vi "Main.vi"() -> ()   [LabVIEW 2025]
doc: "This template is for the Queued Message Handler design pattern.\n\nThe Event Handling Loop generates messages based on user interface actions.\n\nThe Message Handling Loop processes messages generated by the Event Handling Loop, or by other messages. The messages are string values, so new messages can be added easily to the Message Cases case structure in the Message Handling Loop. Each message cluster can also provide an optional value for Message Data, which is a variant that can be converted to whatever message-specific data is required."
uses:
  controls/UI Data.ctl
  support/Message Queue/Enqueue Message (Single).vi
  <vilib>/Utility/file.llb/Write Delimited Spreadsheet (string).vi
  <vilib>/Utility/error.llb/Error Cluster From Error Code.vi
  <vilib>/ErrorRing/Error Ring.xnode
  support/Message Queue/Message Queue.lvlib
  support/User Event - Stop/User Event - Stop.lvlib
  <instrlib>/BK Precision 9200 Series/BK Precision 9200 Series.lvlib
  <instrlib>/Agilent 34970/Agilent 34970.lvlib
panel:
  out "Table":string[][](table)
  out "Current Cycle":u16
  in  "Total Cycles":u16
  in  "Voltage Channel":string
  out "Connected_RELAY":bool caption="Connected_DAQ"
  in  "RELAY CONTROL":refnum<visa-resource-name>
  out "Connected_DAQ":bool
  in  "DAQ970A":refnum<visa-resource-name>
  out "Connected_ps":bool
  in  "POWER SUPPLY":refnum<visa-resource-name>
  out "DAQ_Amps":dbl format="%#_4fA"
  out "DAQ_Volt":dbl format="%#_4fV"
  out "PS_Amps":dbl format="%#_4fA"
  out "PS_Volt":dbl format="%#_4fV"
  out "Status":string
  in  "Start/Stop":enum32{"Item 0", "Item 1"}(radio)=enum."Item 1"
  in  "Exit":bool
  # "DC-DC Short Circuit Durability"
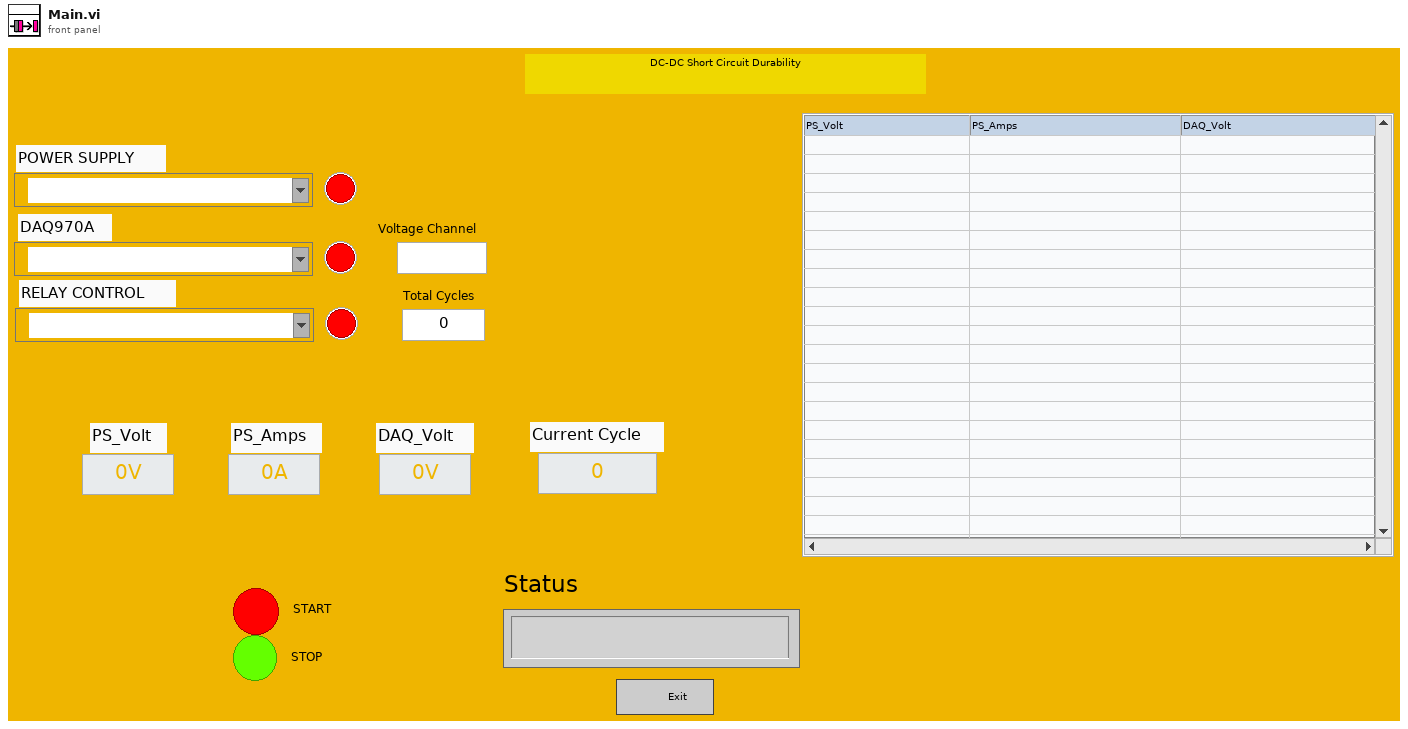
[diagram p1: front panel]
types:
  T1 = typedef "UI Data.ctl" = cluster{"Boolean <Replace Me>":bool, "Status":string, "Cycle Count":u16, "POWER SUPPLY":refnum<visa-resource-name>, "DAQ6510":refnum<visa-resource-name>, "RELAY CONTROL":refnum<visa-resource-name>, "Error Status ":string, "Current Cycle":u16, "Table":string[][], "Data_array":string[], "Started?":bool, "Datapath":path}
  T2 = typedef "Message Queue.lvlib/All Message Queues.ctl" = cluster{"UI":refnum<queue>}
  T3 = enum16{"4 1/2", "5 1/2", "6 1/2", "Least", "Highest", "Default"}
  T4 = cluster{"Timeout Value (10000)":u32, "Baud Rate (57600)":enum16{"1200", "2400", "4800", "9600", "19200", "38400", "57600", "115200"}, "Flow Control (1:XON/XOFF)":enum16{"None", "XON / XOFF", "RTS / CTS", "DTR / DSR"}}
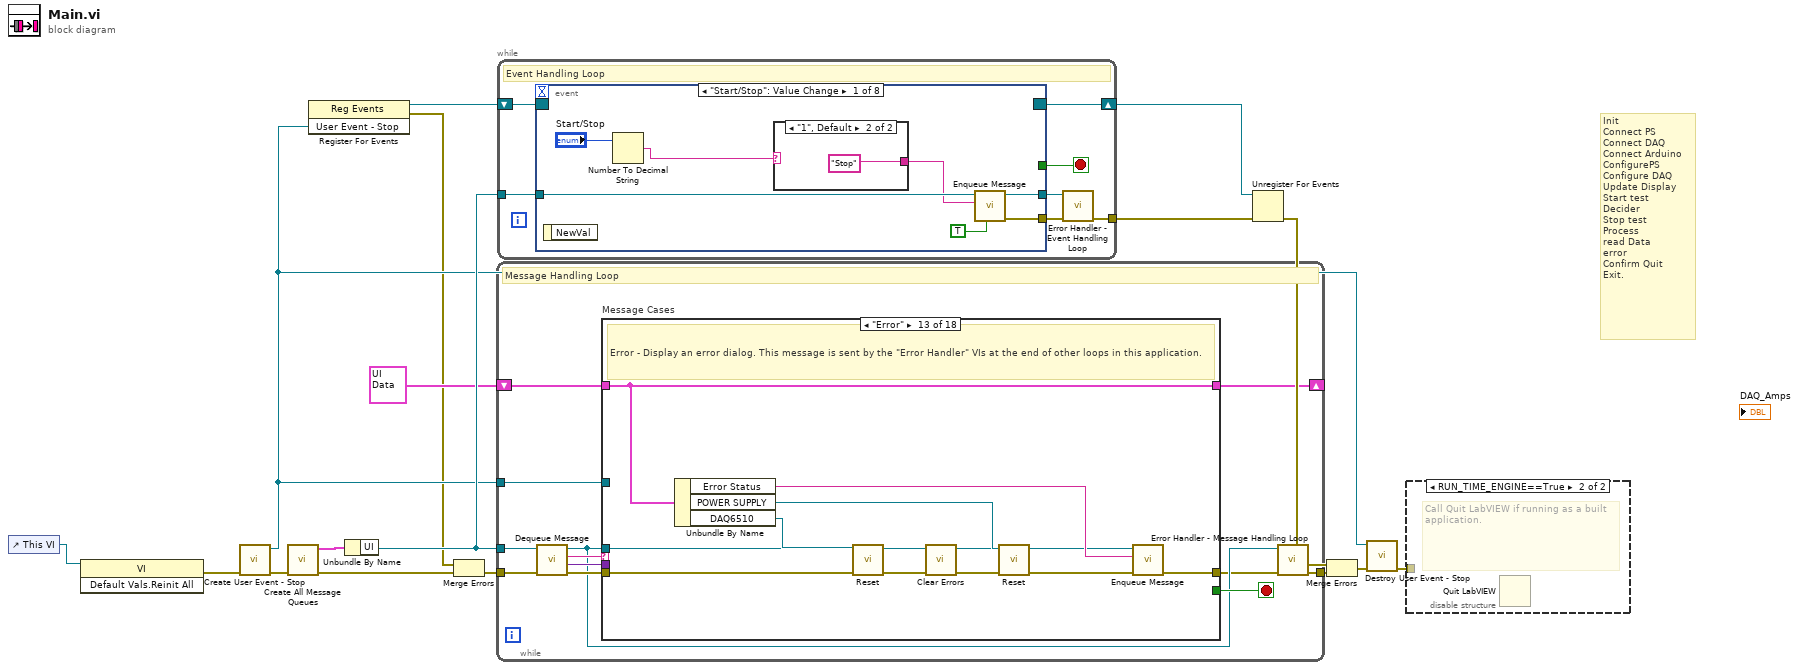
[diagram p0: block diagram]
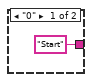
[diagram p3: hidden frame]
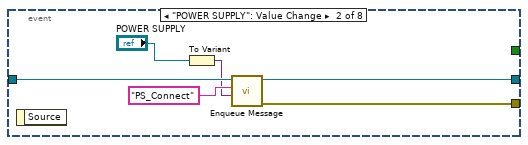
[diagram p4: hidden frame]
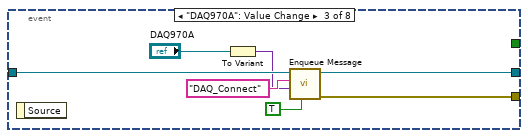
[diagram p5: hidden frame]
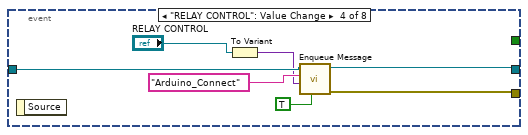
[diagram p6: hidden frame]
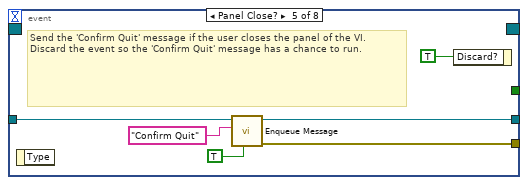
[diagram p7: hidden frame]
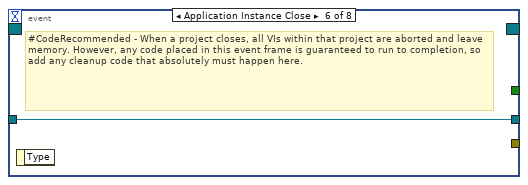
[diagram p8: hidden frame]
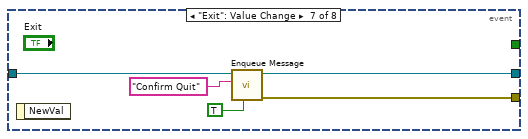
[diagram p9: hidden frame]
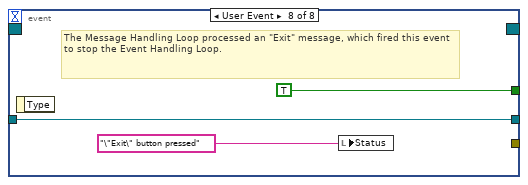
[diagram p10: hidden frame]
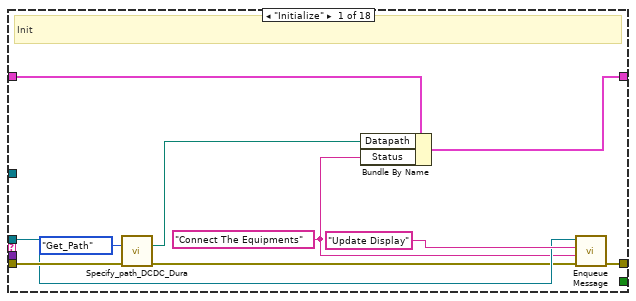
[diagram p11: hidden frame]
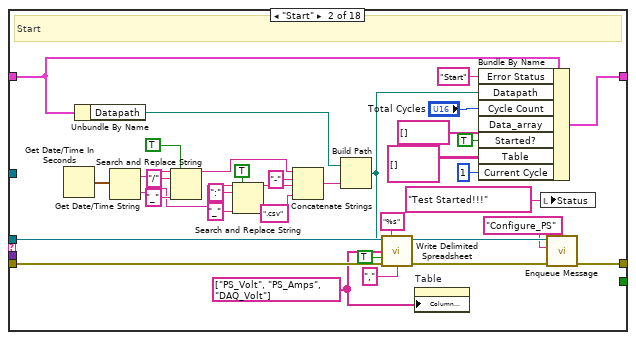
[diagram p12: hidden frame]
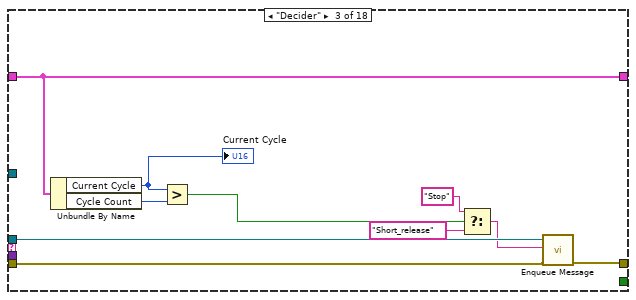
[diagram p13: hidden frame]
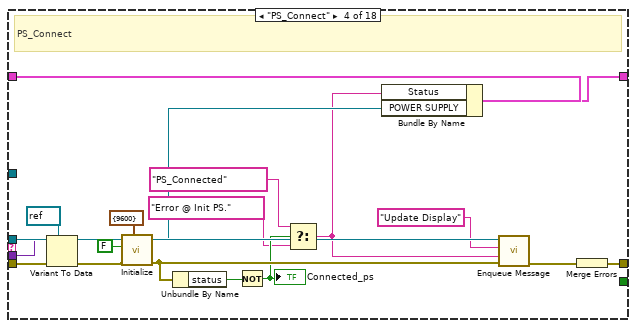
[diagram p14: hidden frame]
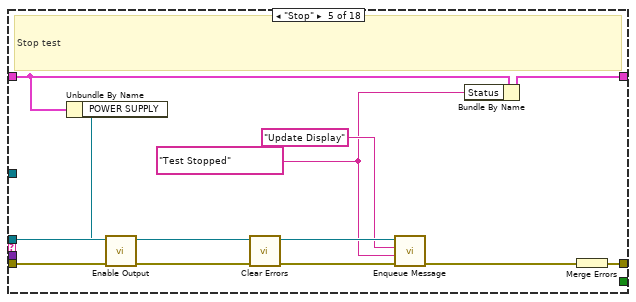
[diagram p15: hidden frame]
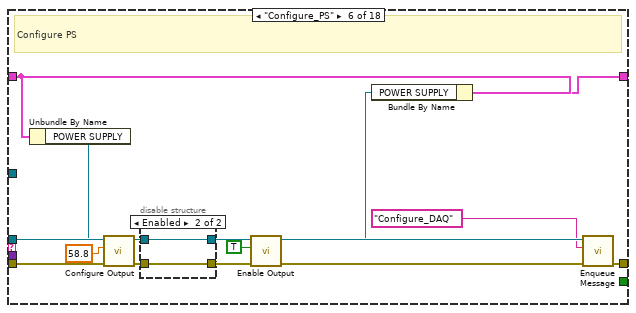
[diagram p16: hidden frame]
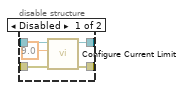
[diagram p17: hidden frame]
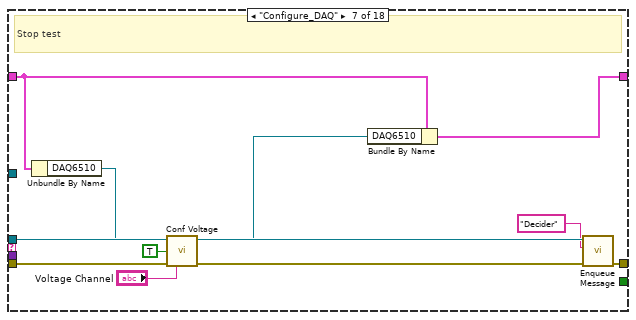
[diagram p18: hidden frame]
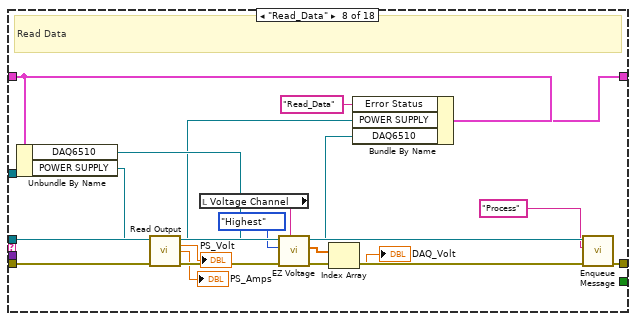
[diagram p19: hidden frame]
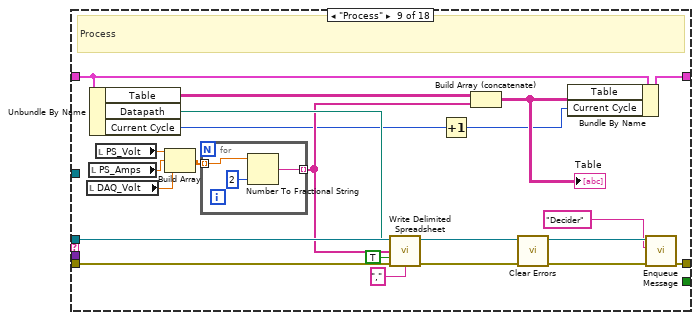
[diagram p20: hidden frame]
diagram:
  # "Init \nConnect PS\nConnect DAQ\nConnect Arduino\nConfigurePS\nConfigure DAQ\nUpdate Display\nStart test\nDecider\nStop test \nProcess \nread Data\nerror\nConfirm Quit\nExit."
  n1 = control-ref of="This VI"() -> (w2:refnum<vi>)
  n2 = invoke class="VI" method="Default Vals.Reinit All"(reference=w2) -> (error out=w1:errorcluster)  [unwired: 2 in, 2 out]
  n3 = call "Create User Event - Stop.vi"("error in (no error)"=w1) -> ("error out"=w13:errorcluster, "User Event - Stop"=w5:refnum<user-event>)  [unwired: 9 in]
  n4 = call "Create All Message Queues.vi"("error in (no error)"=w13) -> ("error out"=w17:errorcluster, "Message Queues out"=w16:T2)  [unwired: 9 in]
  n5 = register-events(w5) -> (reference out=w6:refnum<event-registration>, error out=w3:errorcluster)  [unwired: 2 in]
  n6 = Unbundle By Name(w16) -> ("UI"=w14:refnum<queue>)
  n7 = Merge Errors(w3, w17) -> (w4:errorcluster)
  n8 = while {
    tunnel: w14 -> [w21]
    shift-right: [w28] -> _
    shift-left: T1 {"Boolean <Replace Me>"=FALSE, "Status"="", "Cycle Count"=0, "POWER SUPPLY"="", "DAQ6510"="", "RELAY CONTROL"="", "Error Status "="", "Current Cycle"=0, "Table"=[], "Data_array"=[], "Started?"=FALSE, "Datapath"=path ""} ("Data Cluster") -> [w29]
    tunnel: w5 -> [w26]
    tunnel: w4 -> [w25]
    tunnel: [w19] -> w15
    stop <- w27 stop-if-true
    # "Message Handling Loop"
    n9 = call "Dequeue Message.vi"("error in (no error)"=w25, "Message Queue"=w21) -> ("error out"=w24:errorcluster, "Message Data"=w22:variant, "Message"=w23:string, "dup Message Queue"=w20:refnum<queue>)  [unwired: 6 in]
    n10 = case "Message Cases" shown="\"Error\"" w23 {
      selector: w23 -> [_ _ _ _ _ _ _ _ _ _ _ _ _ _ _ _ _ w303]
      tunnel: w20 -> [w34 w73 w81 w99 w111 w128 w146 w165 w185 w206 w224 _ w232 w255 w265 _ w302 _]
      tunnel: w24 -> [w38 w69 w83 w101 w113 w129 w147 w166 w186 w207 w222 w230 w241 w258 w276 w291 w295 _]
      tunnel: [w39 w70 w82 w102 w114 w126 w144 w163 w183 w204 w226 w231 w234 w257 w275 w289 w298 w304] -> w18
      tunnel: w29 -> [w37 w67 w80 w103 w106 w125 w143 w162 w178 w208 w227 w229 w240 w246 w272 w290 w301 w305]
      tunnel: [w36 w71 w80 w86 w109 w119 w137 w159 w173 w192 w216 w229 w240 w246 w268 w290 w301 w305] -> w28
      tunnel: [_ _ _ _ _ _ _ _ _ _ _ _ _ _ _ _ TRUE _] -> w27
      tunnel: w22 -> [_ _ _ w97 _ _ _ _ _ w201 w220 _ _ _ _ _ w292 _]
      tunnel: w26 -> [_ _ _ _ _ _ _ _ _ _ _ _ _ _ _ _ w297 _]
      frame "Initialize" {
        w33 = "Connect The Equipments" ("Initial Message")
        # "Init"
        n11 = call "Specify_path_DCDC_Dura.vi"("Path_Enum"=enum16{"Find_Path", "Get_Path"}."Get_Path", "error in (no error)"=w38) -> ("DATA"=w30:path, "error out"=w32:errorcluster)  [unwired: 7 in, 5 out]
        n12 = Bundle By Name(cluster=w37, "Datapath"=w30, "Status"=w33) -> (w36:T1)
        n13 = call-poly "Enqueue Message.vi"("error in (no error)"=w32, "Message Data"=w33, "Message"="Update Display", "Message Queue"=w34) -> ("error out"=w39:errorcluster)  [unwired: 6 in, 1 out]
      }
      frame "Start" {
        w43 = string[] ["PS_Volt", "PS_Amps", "DAQ_Volt"]
        # "Start"
        n14 = Get Date/Time In Seconds() -> (seconds since 1Jan1904=w66:timestamp)
        n15 = Unbundle By Name(w67) -> ("Datapath"=w53:path)
        n16 = Get Date/Time String(seconds (now)=w66) -> (date string=w65:string, time string=w62:string)  [unwired: 2 in]
        n17 = Search and Replace String(replace all?=TRUE ("replace all? (F)"), input string=w65, search string="/", replace string="_" ("replace string (\"\")")) -> (result string=w56:string)  [unwired: 4 in, 3 out]
        n18 = Search and Replace String(replace all?=TRUE ("replace all? (F)"), input string=w62, search string=":", replace string="_" ("replace string (\"\")")) -> (result string=w58:string)  [unwired: 4 in, 3 out]
        n19 = Concatenate Strings(w56, "-" ("string"), w58, ".csv" ("string")) -> (w54:string)
        n20 = Build Path(base path=w53, name or relative path=w54) -> (appended path=w52:path)
        n21 = call-poly <vilib>:"Write Delimited Spreadsheet.vi"("file path (dialog if empty)"=w52, "format (%s)"="%s", "1D data"=w43, "append to file? (new file:F)"=TRUE, "error in (no error)"=w69, "delimiter (\\t)"="," ("delimiter (\\t)")) -> ("error out"=w68:errorcluster)  [unwired: 8 in, 1 out]
        n22 = property on="Table" class="Tbl (strict)"("Column Headers[]"=w43) -> ()  [unwired: 2 in, 2 out]
        n23 = Bundle By Name(cluster=w67, "Error Status"="Start", "Datapath"=w52, "Cycle Count"="Total Cycles", "Data_array"=string[] [], "Started?"=TRUE, "Table"=string[][] [], "Current Cycle"=u16 1) -> (w71:T1)
        n24 = local write "Status"("Test Started!!!" ("Status")) -> ()
        n25 = call-poly "Enqueue Message.vi"("error in (no error)"=w68, "Message"="Configure_PS", "Message Queue"=w73) -> ("error out"=w70:errorcluster)  [unwired: 7 in, 1 out]
      }
      frame "Decider" {
        n26 = Unbundle By Name(w80) -> ("Current Cycle"=w74:u16, "Cycle Count"=w79:u16)
        "Current Cycle" <- w74
        n27 = Greater?(x=w74, y=w79) -> (0:w77:bool)
        n28 = Select(t="Stop" ("Message"), s=w77, f="Short_release") -> (s? t:f=w75:string)
        n29 = call-poly "Enqueue Message.vi"("error in (no error)"=w83, "Message"=w75, "Message Queue"=w81) -> ("error out"=w82:errorcluster)  [unwired: 7 in, 1 out]
      }
      frame "PS_Connect" {
        # "PS_Connect"
        n30 = Variant To Data(error in=w101, type=refnum<visa-resource-name> refnum ("POWER SUPPLY"), Variant=w97) -> (data=w94:refnum<visa-resource-name>, error out=w95:errorcluster)
        n31 = call <instrlib>:"Initialize.vi"("Serial Configuration"=cluster{"Baud Rate":u32} {"Baud Rate"=9600}, "error in (no error)"=w95, "ID Query (True)"=FALSE, "VISA resource name"=w94) -> ("error out"=w91:errorcluster, "VISA resource name out"=w85:refnum<visa-resource-name>)  [unwired: 6 in]
        n32 = Unbundle By Name(w91) -> ("status"=w90:bool)
        n33 = Not(x=w90) -> (.not. x?=w89:bool)
        "Connected_ps" <- w89
        n34 = Select(t="PS_Connected" ("\"Do Something\" button pressed"), s=w89, f="Error @ Init PS." ("\"Do Something\" button pressed")) -> (s? t:f=w84:string)
        n35 = Bundle By Name(cluster=w103, "Status"=w84, "POWER SUPPLY"=w85) -> (w86:T1)
        n36 = call-poly "Enqueue Message.vi"("error in (no error)"=w91, "Message Data"=w84, "Message"="Update Display", "Message Queue"=w99) -> ("error out"=w100:errorcluster)  [unwired: 6 in, 1 out]
        n37 = Merge Errors(w100) -> (w102:errorcluster)
      }
      frame "Stop" {
        w108 = "Test Stopped" ("\"Do Something Else\" button pressed")
        # "Stop test"
        n38 = Unbundle By Name(w106) -> ("POWER SUPPLY"=w104:refnum<visa-resource-name>)
        n39 = call <instrlib>:"Enable Output.vi"("error in (no error)"=w113, "VISA resource name"=w104) -> ("error out"=w107:errorcluster)  [unwired: 8 in, 1 out]
        n40 = call <vilib>:"Clear Errors.vi"("error in (no error)"=w107) -> ("error out"=w105:errorcluster)  [unwired: 5 in, 1 out]
        n41 = call-poly "Enqueue Message.vi"("error in (no error)"=w105, "Message Data"=w108, "Message"="Update Display", "Message Queue"=w111) -> ("error out"=w112:errorcluster)  [unwired: 6 in, 1 out]
        n42 = Bundle By Name(cluster=w106, "Status"=w108) -> (w109:T1)
        n43 = Merge Errors(w112) -> (w114:errorcluster)
      }
      frame "Configure_PS" {
        # "Configure PS"
        n44 = Unbundle By Name(w125) -> ("POWER SUPPLY"=w123:refnum<visa-resource-name>)
        n45 = call <instrlib>:"Configure Output.vi"("error in (no error)"=w129, "Voltage Level (0.0 V)"=58.8, "VISA resource name"=w123) -> ("error out"=w124:errorcluster, "VISA resource name out"=w120:refnum<visa-resource-name>)  [unwired: 7 in]
        n46 = disable-structure shown="Enabled" {
          disable-tunnel: w124 -> [w134 w136]
          disable-tunnel: [w133 w136] -> w121
          disable-tunnel: w120 -> [w132 w135]
          disable-tunnel: [w130 w135] -> w117
          frame Disabled {
            n47 = call <instrlib>:"Configure Current Limit.vi"("error in (no error)"=w134, "Current Limit (0.0 A)"=9.0, "VISA resource name"=w132) -> ("error out"=w133:errorcluster, "VISA resource name out"=w130:refnum<visa-resource-name>)  [unwired: 7 in]
          }
          frame Enabled {
          }
        }
        n48 = call <instrlib>:"Enable Output.vi"("error in (no error)"=w121, "Enable Output (F: False)"=TRUE, "VISA resource name"=w117) -> ("error out"=w118:errorcluster, "VISA resource name out"=w116:refnum<visa-resource-name>)  [unwired: 7 in]
        n49 = Bundle By Name(cluster=w125, "POWER SUPPLY"=w116) -> (w119:T1)
        n50 = call-poly "Enqueue Message.vi"("error in (no error)"=w118, "Message"="Configure_DAQ", "Message Queue"=w128) -> ("error out"=w126:errorcluster)  [unwired: 7 in, 1 out]
      }
      frame "Configure_DAQ" {
        # "Stop test"
        n51 = Unbundle By Name(w143) -> ("DAQ6510"=w141:refnum<visa-resource-name>)
        n52 = call <instrlib>:"Conf Voltage.vi"("VISA Resource Name"=w141, "Autorange? (F:Off)"=TRUE, "error in (no error)"=w147, "Channel List (empty)"="Voltage Channel") -> ("VISA Resource Name Out"=w138:refnum<visa-resource-name>, "error out"=w142:errorcluster)  [unwired: 9 in, 1 out]
        n53 = Bundle By Name(cluster=w143, "DAQ6510"=w138) -> (w137:T1)
        n54 = call-poly "Enqueue Message.vi"("error in (no error)"=w142, "Message"="Decider", "Message Queue"=w146) -> ("error out"=w144:errorcluster)  [unwired: 7 in, 1 out]
      }
      frame "Read_Data" {
        # "Read Data"
        n55 = Unbundle By Name(w162) -> ("DAQ6510"=w155:refnum<visa-resource-name>, "POWER SUPPLY"=w156:refnum<visa-resource-name>)
        n56 = call <instrlib>:"Read Output.vi"("VISA resource name"=w156, "error in (no error)"=w166) -> ("VISA resource name out"=w154:refnum<visa-resource-name>, "Actual Voltage Level (V)"=→"PS_Volt":dbl, "Actual Current Level (A)"=→"PS_Amps":dbl, "error out"=w157:errorcluster)  [unwired: 9 in, 1 out]
        n57 = local read "Voltage Channel"() -> (w158:string)
        n58 = call <instrlib>:"EZ Voltage.vi"("Scan List (empty)"=w158, "error in (no error)"=w157, "Resolution (5:Default)"=T3."Highest", "VISA Resource Name"=w155) -> ("error out"=w161:errorcluster, "Output Array"=w152:dbl[], "VISA Resource Name Out"=w160:refnum<visa-resource-name>)  [unwired: 5 in]
        n59 = Index Array(array=w152) -> (element=→"DAQ_Volt":dbl)  [unwired: 1 in]
        n60 = Bundle By Name(cluster=w162, "Error Status"="Read_Data", "POWER SUPPLY"=w154, "DAQ6510"=w160) -> (w159:T1)
        n61 = call-poly "Enqueue Message.vi"("error in (no error)"=w161, "Message"="Process", "Message Queue"=w165) -> ("error out"=w163:errorcluster)  [unwired: 7 in, 1 out]
      }
      frame "Process" {
        # "Process"
        n62 = local read "DAQ_Volt"() -> (w182:dbl)
        n63 = local read "PS_Amps"() -> (w181:dbl)
        n64 = Unbundle By Name(w178) -> ("Table"=w172:string[][], "Datapath"=w176:path, "Current Cycle"=w169:u16)
        n65 = local read "PS_Volt"() -> (w180:dbl)
        n66 = Build Array(w180, w181, w182) -> (w179:dbl[])
        n67 = for {
          tunnel: w179 -> [w189] mode=indexing
          tunnel: [w187] -> w171 mode=indexing
          n68 = Number To Fractional String(number=w189, precision (6)=i16 2) -> (F-format string=w187:string)  [unwired: 2 in]
        }
        n69 = call-poly <vilib>:"Write Delimited Spreadsheet.vi"("file path (dialog if empty)"=w176, "1D data"=w171, "append to file? (new file:F)"=TRUE, "error in (no error)"=w186, "delimiter (\\t)"="," ("delimiter (\\t)")) -> ("error out"=w177:errorcluster)  [unwired: 9 in, 1 out]
        n70 = Increment(x=w169) -> (x+1=w168:u16)
        n71 = Build Array (concatenate)(w172, w171) -> (w170:string[][])
        "Table" <- w170
        n72 = call <vilib>:"Clear Errors.vi"("error in (no error)"=w177) -> ("error out"=w167:errorcluster)  [unwired: 5 in, 1 out]
        n73 = Bundle By Name(cluster=w178, "Table"=w170, "Current Cycle"=w168) -> (w173:T1)
        n74 = call-poly "Enqueue Message.vi"("error in (no error)"=w167, "Message"="Decider", "Message Queue"=w185) -> ("error out"=w183:errorcluster)  [unwired: 7 in, 1 out]
      }
      frame "DAQ_Connect" {
        # "DAQ_Connection"
        n75 = Variant To Data(error in=w207, type=refnum<visa-resource-name> refnum ("POWER SUPPLY"), Variant=w201) -> (data=w199:refnum<visa-resource-name>, error out=w198:errorcluster)
        n76 = call <instrlib>:"Initialize.vi"("VISA Resource Name"=w199, "ID Query (T: Check)"=FALSE, "Serial Port Configuration"=T4 {"Timeout Value (10000)"=1000, "Baud Rate (57600)"=enum."9600", "Flow Control (1:XON/XOFF)"=enum."None"}, "error in (no error)"=w198) -> ("VISA Resource Name Out"=w191:refnum<visa-resource-name>, "error out"=w195:errorcluster)  [unwired: 10 in]
        n77 = Unbundle By Name(w195) -> ("status"=w194:bool)
        n78 = Not(x=w194) -> (.not. x?=w193:bool)
        "Connected_DAQ" <- w193
        n79 = Select(t="DAQ_Connected" ("\"Do Something\" button pressed"), s=w193, f="Error @ DAQ_Connect" ("\"Do Something\" button pressed")) -> (s? t:f=w190:string)
        n80 = Bundle By Name(cluster=w208, "DAQ6510"=w191, "Status"=w190) -> (w192:T1)
        n81 = call-poly "Enqueue Message.vi"("error in (no error)"=w195, "Message Data"=w190, "Message"="Update Display", "Message Queue"=w206) -> ("error out"=w204:errorcluster)  [unwired: 6 in, 1 out]
      }
      frame "Arduino_Connect" {
        # "Arduino Connect"
        n82 = Variant To Data(error in=w222, type=refnum<visa-resource-name> refnum ("POWER SUPPLY"), Variant=w220) -> (data=w218:refnum<visa-resource-name>, error out=w221:errorcluster)
        n83 = call "Arduino_DCDC_Durability.vi"("error out"=w221, "Enum"=enum16{"Init", "Poll", "Read", "Write", "Exit"}."Init", "VISA resource name"=w218) -> ("error out 2"=w214:errorcluster, "VISA out"=w215:refnum<visa-resource-name>)  [unwired: 6 in, 1 out]
        n84 = Unbundle By Name(w214) -> ("status"=w213:bool)
        n85 = Not(x=w213) -> (.not. x?=w212:bool)
        "Connected_RELAY" <- w212
        n86 = Select(t="Arduino_Connected" ("\"Do Something\" button pressed"), s=w212, f="Error @ Arduino Connect" ("\"Do Something\" button pressed")) -> (s? t:f=w209:string)
        n87 = Bundle By Name(cluster=w227, "RELAY CONTROL"=w215, "Status"=w209) -> (w216:T1)
        n88 = call-poly "Enqueue Message.vi"("error in (no error)"=w214, "Message Data"=w209, "Message"="Update Display", "Message Queue"=w224) -> ("error out"=w225:errorcluster)  [unwired: 6 in, 1 out]
        n89 = Merge Errors(w225) -> (w226:errorcluster)
      }
      frame "Update Display" {
        # "Update Display - Convert the message data to a string to display in the Data Display indicator."
        n90 = Unbundle By Name(w229) -> ("Status"=→"Status":string)
        n91 = Merge Errors(w230) -> (w231:errorcluster)
      }
      frame "Error" {
        # "Error - Display an error dialog. This message is sent by the \"Error Handler\" VIs at the end of other loops in this application."
        n92 = Unbundle By Name(w240) -> ("Error Status"=w233:string, "POWER SUPPLY"=w236:refnum<visa-resource-name>, "DAQ6510"=w238:refnum<visa-resource-name>)
        n93 = call <instrlib>:"Reset.vi"("VISA Resource Name"=w238, "error in (no error)"=w241) -> ("error out"=w239:errorcluster)  [unwired: 12 in, 1 out]
        n94 = call <vilib>:"Clear Errors.vi"("error in (no error)"=w239) -> ("error out"=w237:errorcluster)  [unwired: 5 in, 1 out]
        n95 = call <instrlib>:"Reset.vi"("error in (no error)"=w237, "VISA resource name"=w236) -> ("error out"=w235:errorcluster)  [unwired: 8 in, 1 out]
        n96 = call-poly "Enqueue Message.vi"("error in (no error)"=w235, "Message"=w233, "Message Queue"=w232) -> ("error out"=w234:errorcluster)  [unwired: 7 in, 1 out]
      }
      frame "Confirm Quit" {
        # "Confirm Quit - Message that can confirm whether or not the user wants to exit the application."
        n97 = Unbundle By Name(w246) -> ("POWER SUPPLY"=w245:refnum<visa-resource-name>, "DAQ6510"=w244:refnum<visa-resource-name>, "RELAY CONTROL"=w243:refnum<visa-resource-name>)
        n98 = call <instrlib>:"Close.vi"("error in (no error)"=w258, "VISA resource name"=w245) -> ("error out"=w252:errorcluster)  [unwired: 9 in]
        n99 = call <vilib>:"Clear Errors.vi"("error in (no error)"=w252) -> ("error out"=w250:errorcluster)  [unwired: 5 in, 1 out]
        n100 = call <instrlib>:"Close.vi"("VISA Resource Name"=w244, "error in (no error)"=w250) -> ("error out"=w251:errorcluster)  [unwired: 13 in]
        n101 = call <vilib>:"Clear Errors.vi"("error in (no error)"=w251) -> ("error out"=w249:errorcluster)  [unwired: 5 in, 1 out]
        n102 = call "Arduino_DCDC_Durability.vi"("error out"=w249, "Enum"=enum16{"Init", "Poll", "Read", "Write", "Exit"}."Exit", "VISA resource name"=w243) -> ("error out 2"=w248:errorcluster)  [unwired: 6 in, 2 out]
        n103 = call <vilib>:"Clear Errors.vi"("error in (no error)"=w248) -> ("error out"=w242:errorcluster)  [unwired: 5 in, 1 out]
        n104 = call-poly "Enqueue Message.vi"("Priority Message? (F)"=TRUE, "error in (no error)"=w242, "Message"="Exit", "Message Queue"=w255) -> ("error out"=w256:errorcluster)  [unwired: 6 in, 1 out]
        n105 = Merge Errors(w256) -> (w257:errorcluster)
      }
      frame "Short_release" {
        # "To short and release the relay"
        n106 = Unbundle By Name(w272) -> ("RELAY CONTROL"=w271:refnum<visa-resource-name>)
        n107 = flat-sequence {
          tunnel: w276 -> [w282]
          tunnel: w271 -> [w281]
          tunnel: [w278] -> w260
          tunnel: [w277] -> w259
          tunnel: [w284] -> w263
          tunnel: [w285] -> w269
          tunnel: w260 -> [w285]
          tunnel: w259 -> [w284]
          frame #0 {
            n108 = call "Arduino_DCDC_Durability.vi"("DO's"=string[] ["1"], "error out"=w282, "Enum"=enum16{"Init", "Poll", "Read", "Write", "Exit"}."Write", "VISA resource name"=w281) -> ("error out 2"=w277:errorcluster, "VISA out"=w278:refnum<visa-resource-name>)  [unwired: 5 in, 1 out]
          }
          frame #1 {
            n109 = Wait (ms)(milliseconds to wait=u32 4000) -> ()  [unwired: 1 out]
          }
        }
        n110 = call "Arduino_DCDC_Durability.vi"("DO's"=string[] ["5"], "Enum"=enum16{"Init", "Poll", "Read", "Write", "Exit"}."Write", "VISA resource name"=w269) -> ("VISA out"=w267:refnum<visa-resource-name>)  [unwired: 6 in, 2 out]
        n111 = flat-sequence {
          tunnel: w265 -> [w288]
          tunnel: [w288] -> w264
          tunnel: w263 -> [w286]
          tunnel: [w286] -> w262
          frame #0 {
            n112 = Wait (ms)(milliseconds to wait=u32 3000) -> ()  [unwired: 1 out]
          }
        }
        n113 = Bundle By Name(cluster=w272, "RELAY CONTROL"=w267, "Error Status"="Short_release") -> (w268:T1)
        n114 = call-poly "Enqueue Message.vi"("Priority Message? (F)"=TRUE, "error in (no error)"=w262, "Message"="Read_Data", "Message Queue"=w264) -> ("error out"=w275:errorcluster)  [unwired: 6 in, 1 out]
      }
      frame "---Copy This Frame---" {
        # "Duplicate this frame when creating new messages.  Change this comment in the duplicated frame to describe this message."
        n115 = Merge Errors(w291) -> (w289:errorcluster)
      }
      frame "Exit" {
        # "Stop the VI"
        # "Release the message queue reference"
        # "#CodeNeeded - Add any required cleanup code here. Note that if 'Exit' was called as a result of an error, an error dialog will be displayed. Add any custom error handling for an 'Exit' condition here as well."
        # "Exit - Exit the application."
        n116 = Variant To Data(type=errorcluster {"status"=FALSE, "code"=0, "source"=""} ("error constant"), Variant=w292) -> (data=w293:errorcluster)  [unwired: 1 in, 1 out]
        n117 = call <vilib>:"Simple Error Handler.vi"("error in (no error)"=w293) -> ()  [unwired: 4 in, 5 out]
        n118 = call "Fire User Event - Stop.vi"("User Event - Stop"=w297) -> ("error out"=w296:errorcluster)  [unwired: 10 in]
        n119 = Release Queue(queue=w302, error in (no error)=w295) -> (error out=w299:errorcluster)  [unwired: 1 in, 2 out]
        n120 = Merge Errors(w296, w299) -> (w298:errorcluster)
      }
      frame Default {
        # "'Default' case only runs if there is a message that isn't defined in any of the other cases.  Output a programming error."
        n121 = xnode "Error Ring"("parameter 0"=w303) -> ("error out"=w304:errorcluster)
      }
    }
    n122 = call "Error Handler - Message Handling Loop.vi"("error in (no error)"=w18, "Message Queue"=w20) -> ("dup error in"=w19:errorcluster)  [unwired: 8 in, 1 out]
  }
  n123 = while {
    tunnel: w14 -> [w319]
    shift-right: [w317] -> w10
    shift-left: w6 -> [w318]
    tunnel: [w313] -> w7
    stop <- w315 stop-if-true
    # "Event Handling Loop"
    n124 = event shown="[0] \"Start/Stop\": Value Change" {
      selector: w318 -> [_ _ _ _ _ _ _ _]
      dyn-events: [_ _ _ _ _ _ _ _] -> w317
      timeout: _ -> [_ _ _ _ _ _ _ _]
      tunnel: [_ _ _ _ _ _ _ TRUE ("Discard?")] -> w315
      tunnel: w319 -> [w326 w334 w338 w345 w353 w355 w360 w363]
      tunnel: [w324 w331 w339 w346 w352 _ w359 _] -> w316
      tunnel: [w325 w333 w337 w344 w351 w355 w358 w363] -> w314
      event "Start/Stop": Value Change {
        n125 = event-data() -> ()  [unwired: 1 in, 1 out]
        n126 = Number To Decimal String(number="Start/Stop") -> (decimal integer string=w322:string)  [unwired: 1 in]
        n127 = case shown="\"1\", Default" w322 {
          tunnel: ["Start" "Stop"] -> w321
          frame "0" {
          }
          frame "1", Default {
          }
        }
        n128 = call-poly "Enqueue Message.vi"("Priority Message? (F)"=TRUE, "Message"=w321, "Message Queue"=w326) -> ("error out"=w324:errorcluster, "dup Message Queue"=w325:refnum<queue>)  [unwired: 7 in]
      }
      event "POWER SUPPLY": Value Change {
        n129 = event-data() -> ()  [unwired: 1 in, 1 out]
        n130 = To Variant(anything="POWER SUPPLY") -> (Variant=w329:variant)
        n131 = call-poly "Enqueue Message.vi"("Message Data"=w329, "Message"="PS_Connect", "Message Queue"=w334) -> ("error out"=w331:errorcluster, "dup Message Queue"=w333:refnum<queue>)  [unwired: 7 in]
      }
      event "DAQ970A": Value Change {
        n132 = event-data() -> ()  [unwired: 1 in, 1 out]
        n133 = To Variant(anything="DAQ970A") -> (Variant=w335:variant)
        n134 = call-poly "Enqueue Message.vi"("Priority Message? (F)"=TRUE, "Message Data"=w335, "Message"="DAQ_Connect", "Message Queue"=w338) -> ("error out"=w339:errorcluster, "dup Message Queue"=w337:refnum<queue>)  [unwired: 6 in]
      }
      event "RELAY CONTROL": Value Change {
        n135 = event-data() -> ()  [unwired: 1 in, 1 out]
        n136 = To Variant(anything="RELAY CONTROL") -> (Variant=w342:variant)
        n137 = call-poly "Enqueue Message.vi"("Priority Message? (F)"=TRUE, "Message Data"=w342, "Message"="Arduino_Connect", "Message Queue"=w345) -> ("error out"=w346:errorcluster, "dup Message Queue"=w344:refnum<queue>)  [unwired: 6 in]
      }
      event Panel Close? {
        # "Send the 'Confirm Quit' message if the user closes the panel of the VI. Discard the event so the 'Confirm Quit' message has a chance to run."
        n138 = event-data() -> ()  [unwired: 1 in, 1 out]
        n139 = call-poly "Enqueue Message.vi"("Priority Message? (F)"=TRUE, "Message"="Confirm Quit", "Message Queue"=w353) -> ("error out"=w352:errorcluster, "dup Message Queue"=w351:refnum<queue>)  [unwired: 7 in]
        n140 = event-data("Discard?"=TRUE) -> ()  [unwired: 1 in, 1 out]
      }
      event Application Instance Close {
        # "#CodeRecommended - When a project closes, all VIs within that project are aborted and leave memory. However, any code placed in this event frame is guaranteed to run to completion, so add any cleanup code that absolutely must happen here."
        n141 = event-data() -> ()  [unwired: 1 in, 1 out]
      }
      event "Exit": Value Change {
        n142 = event-data() -> ()  [unwired: 1 in, 1 out]
        n143 = call-poly "Enqueue Message.vi"("Priority Message? (F)"=TRUE, "Message"="Confirm Quit", "Message Queue"=w360) -> ("error out"=w359:errorcluster, "dup Message Queue"=w358:refnum<queue>)  [unwired: 7 in]
      }
      event User Event {
        # "The Message Handling Loop processed an \"Exit\" message, which fired this event to stop the Event Handling Loop."
        n144 = event-data() -> ()  [unwired: 1 in, 1 out]
        n145 = local write "Status"("\"Exit\" button pressed" ("VI Stopped")) -> ()
      }
    }
    n146 = call "Error Handler - Event Handling Loop.vi"("error in (no error)"=w316, "Message Queue"=w314) -> ("dup error in"=w313:errorcluster)  [unwired: 8 in, 1 out]
  }
  n147 = Unregister For Events(event registration refnum=w10, error in=w7) -> (error out=w11:errorcluster)
  n148 = Merge Errors(w11, w15) -> (w12:errorcluster)
  n149 = call "Destroy User Event - Stop.vi"("error in (no error)"=w12, "User Event - Stop"=w5) -> ("error out"=w8:errorcluster)  [unwired: 9 in]
  n150 = disable-structure shown="RUN_TIME_ENGINE==True" {
    disable-tunnel: w8 -> [_ _]
    frame condition #0 (active) {
    }
    frame condition #1 {
      # "Call Quit LabVIEW if running as a built application."
      n151 = Quit LabVIEW() -> ()  [unwired: 1 in]
    }
  }
